vi "Declare Dependency.vi"(6 "Shared Resource":bool, 8 "error in (no error)":errorcluster, 9 "Name":string, 10 "Dependency":refnum<class "SMO.lvclass">, 11 "SMO in":refnum<class "SMO.lvclass">) -> (0 "error out":errorcluster, 1 "Unique Name":string, 2 "Dependency out":refnum<class "SMO.lvclass">, 3 "SMO out":refnum<class "SMO.lvclass">)   [LabVIEW 2021, in "smo.lvlib" / "SMO.lvclass"]
uses:
  SMO.lvclass
  SMO.lvclass/SMO.ctl
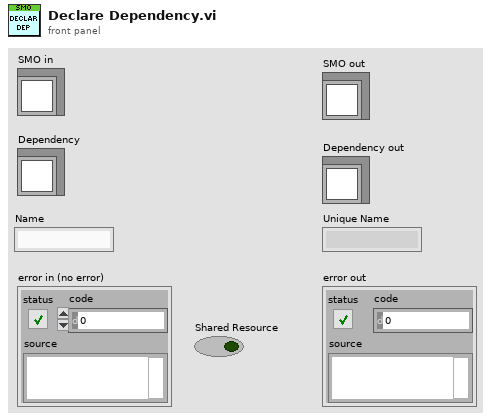
[diagram p1: front panel]
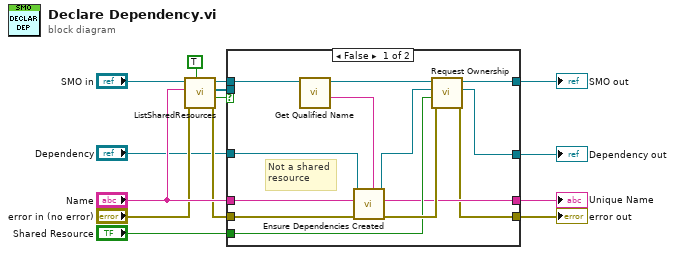
[diagram p0: block diagram]
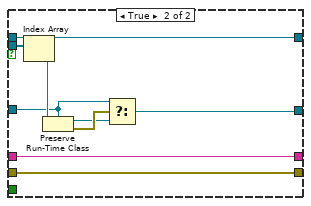
[diagram p2: hidden frame]
diagram:
  n1 = call "ListSharedResources.vi"("exact name? (F: regex)"=TRUE, "error in (no error)"="error in (no error)", "Filter (regex|name)"="Name", "SMO in"="SMO in") -> ("error out"=w11:errorcluster, "resources found?"=w7:bool, "Shared Resources"=w4:refnum<class "SMO.lvclass">[], "SMO out"=w5:refnum<class "SMO.lvclass">)  [unwired: 4 in]
  n2 = case shown="False" w7 {
    tunnel: w4 -> [_ w36]
    tunnel: w5 -> [w17 w35]
    tunnel: [w26 w35] -> w6
    tunnel: [w25 w31] -> w8
    tunnel: "Dependency" -> [w21 w30]
    tunnel: "Name" -> [w27 w28]
    tunnel: w11 -> [w24 w29]
    tunnel: [w18 w29] -> w12
    tunnel: "Shared Resource" -> [w22 _]
    tunnel: [w19 w28] -> w1
    frame False {
      # "Not a shared\nresource"
      n3 = call "Get Qualified Name.vi"("SMO"=w17) -> ("Reserved Qualified Name"=w15:string, "SMO out"=w16:refnum<class "SMO.lvclass">)  [unwired: 7 in, 2 out]
      n4 = call "Ensure Dependencies Created.vi"("Owner Qualified Name"=w15, "error in (no error)"=w24, "Dependency Name"=w27, "SMO in"=w21) -> ("error out"=w23:errorcluster, "Unique Dependency name"=w19:string, "SMO out"=w20:refnum<class "SMO.lvclass">)  [unwired: 5 in]
      n5 = call "Request Ownership.vi"("error in (no error)"=w23, "Shared Resource"=w22, "Dependency"=w20, "SMO in"=w16) -> ("error out"=w18:errorcluster, "Dependency out"=w25:refnum<class "SMO.lvclass">, "SMO out"=w26:refnum<class "SMO.lvclass">)  [unwired: 5 in]
    }
    frame True {
      n6 = Index Array(array=w36) -> (element=w34:refnum<class "SMO.lvclass">)  [unwired: 1 in]
      n7 = Preserve Run-Time Class(object in=w34, 2:w30) -> (object out=w32:refnum<class "SMO.lvclass">, error out=w33:errorcluster)  [unwired: 1 in]
      n8 = Select(t=w30, s=w33, f=w32) -> (s? t:f=w31:refnum<class "SMO.lvclass">)
    }
  }
  "error out" <- w12
  "Dependency out" <- w8
  "SMO out" <- w6
  "Unique Name" <- w1
